vi "Gauge.vi"(5 "Tag Values":string[](array[string]), 7 "Tags":string[](array[string]), 8 "error in (no error)":errorcluster, 9 "Metric Value":dbl, 10 "Metric Name":string, 11 "StatD Interface in":refnum<class "StatD Interface.lvclass">) -> (0 "error out":errorcluster, 3 "StatD Interface out":refnum<class "StatD Interface.lvclass">)   [LabVIEW 2011, in "StatD Interface.lvclass"]
doc: "Record the value of a gauge."
uses:
  StatD Interface.lvclass
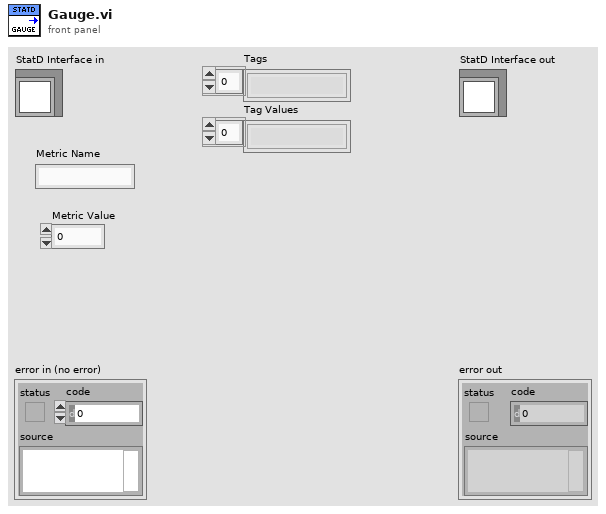
[diagram p1: front panel]
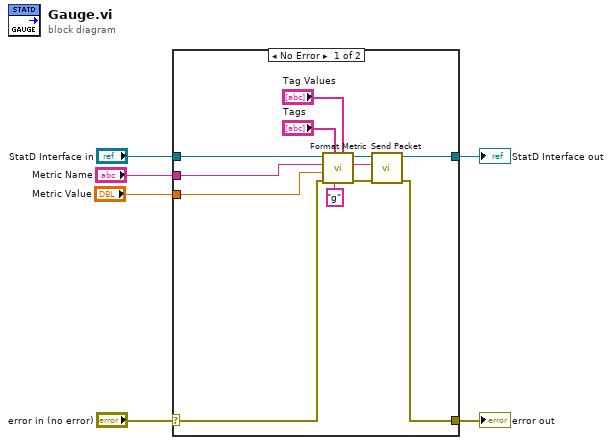
[diagram p0: block diagram]
diagram:
  n1 = case shown="No Error" "error in (no error)" {
    selector: "error in (no error)" -> [w7 w20]
    tunnel: [w17 w20] -> w5
    tunnel: [w18 w19] -> w3
    tunnel: "StatD Interface in" -> [w13 w19]
    tunnel: "Metric Value" -> [w9 _]
    tunnel: "Metric Name" -> [w8 _]
    frame No Error {
      n2 = call "Format Metric.vi"("Tag Values"="Tag Values", "Metric Type"="g", "Tags"="Tags", "error in (no error)"=w7, "Metric Value"=w9, "Metric Name"=w8, "StatD Interface in"=w13) -> ("error out"=w15:errorcluster, "Packet"=w14:string, "StatD Interface out"=w16:refnum<class "StatD Interface.lvclass">)  [unwired: 2 in]
      n3 = call "Send Packet.vi"("error in (no error)"=w15, "Packet"=w14, "StatD Interface in"=w16) -> ("error out"=w17:errorcluster, "StatD Interface out"=w18:refnum<class "StatD Interface.lvclass">)  [unwired: 7 in]
    }
    frame Error {
    }
  }
  "error out" <- w5
  "StatD Interface out" <- w3
